vi "NanoStep WaitMess.vi"(8 "error in":errorcluster, 10 "Abort Ref":refnum<vi>, 11 "Stop Ref":refnum<vi>) -> (0 "error out":errorcluster)   [LabVIEW 2010]
uses:
  <userlib>/GenProg/WritebyRefBool.vi
panel:
  in  "Annuler":bool
  # "Veuiller patienter pendant l'initialisation de l'axe moteur NanoStep"
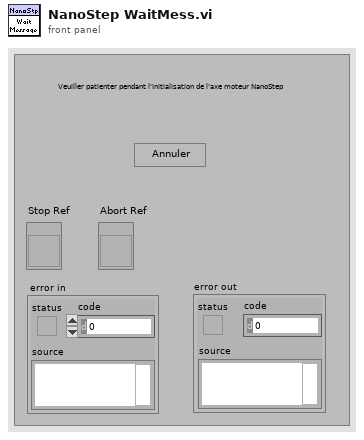
[diagram p1: front panel]
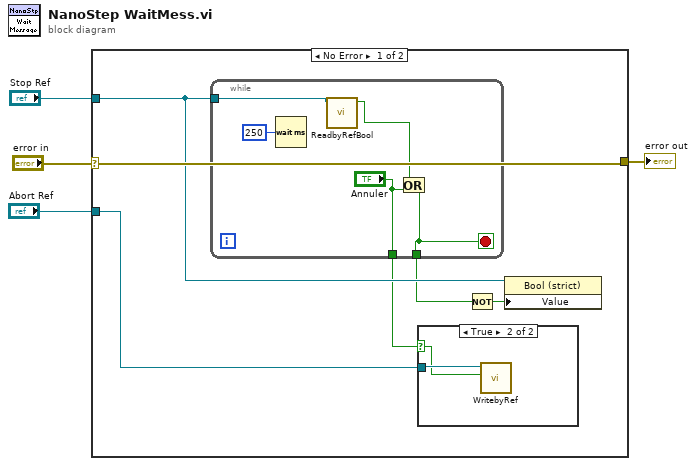
[diagram p0: block diagram]
diagram:
  n1 = case shown="No Error" "error in" {
    selector: "error in" -> [w10 w18]
    tunnel: [w10 w18] -> w3
    tunnel: "Stop Ref" -> [w9 _]
    tunnel: "Abort Ref" -> [w5 _]
    frame No Error {
      n2 = while {
        tunnel: w9 -> [w15]
        tunnel: [w16] -> w8
        tunnel: ["Annuler"] -> w6
        stop <- w16 stop-if-true
        n3 = Wait (ms)(milliseconds to wait=u32 250 ("attente (ms)")) -> ()  [unwired: 1 out]
        n4 = call <userlib>:"ReadbyRefBool.vi"("Control Ref"=w15) -> ("Valeur"=w14:bool)  [unwired: 9 in, 1 out]
        n5 = Or(x=w14, y="Annuler") -> (x .or. y?=w16:bool)
      }
      n6 = case shown="True" w6 {
        selector: w6 -> [_ w11]
        tunnel: w5 -> [_ w12]
        frame False {
        }
        frame True {
          n7 = call-poly <userlib>:"WritebyRef.vi"("Valeur"=w11, "Control Ref"=w12) -> ()  [unwired: 9 in, 1 out]
        }
      }
      n8 = Not(x=w8) -> (.not. x?=w7:bool)
      n9 = property class="Bool (strict)"(reference=w9, "Value"=w7) -> ()  [unwired: 1 in, 2 out]
    }
    frame Error {
    }
  }
  "error out" <- w3
